vi "Pre Launch Init.vi"(11 "CO2 Actor in":refnum<class "CO2 Actor.lvclass">) -> (0 "error out":errorcluster, 3 "CO2 Actor out":refnum<class "CO2 Actor.lvclass">)   [LabVIEW 2015, in "cRIO-Carbondioxide.lvlib" / "CO2-Actor.lvlib" / "CO2 Actor.lvclass"]
doc: "(<B>Filename</B>: Actor Framework.lvlib:Actor.lvclass:Pre Launch Init.vi)\n\nDefines behavior that occurs after the Launch Actor method is invoked but before the actor's Actor Core method begins running.\n\nThe Pre Launch Init method is guaranteed to finish before the Launch Actor method returns to its caller and before the actor itself receives any messages. Any references that the Pre Launch Init method obtains are guaranteed to have the same lifetime as the actor itself. Any errors that the Pre Launch Init method returns will abort the launch.\n\nBy default, this method does nothing. A descendant class may override it to define behavior."
uses:
  CO2 Actor.lvclass
  cRIO-CO2/Debugger.ctl
  CO2 Actor.lvclass/CO2 Actor.ctl
  <vilib>/ActorFramework/Actor/Actor.lvclass/Actor.ctl
  <vilib>/ActorFramework/Message Enqueuer/Message Enqueuer.lvclass/Message Enqueuer.ctl
  <vilib>/ActorFramework/Message Enqueuer/Init from Existing Queue.vi
  <vilib>/ActorFramework/Message Enqueuer/Enqueue.vi
  <vilib>/ActorFramework/Message Priority Queue/Priority Enqueue.vi
  CO2 Actor Messages/Register Self Msg/Register Self Msg.lvclass
  <vilib>/ActorFramework/Message Enqueuer/Message Enqueuer.lvclass
  <vilib>/ActorFramework/Actor/Actor.lvclass
  cRIO-CO2/cRIO-CO2.lvclass
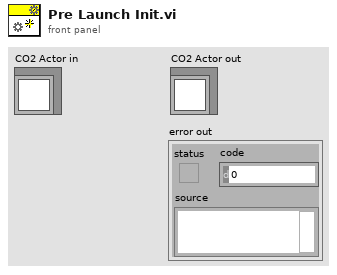
[diagram p1: front panel]
types:
  T1 = typedef "cRIO-Carbondioxide.lvlib/cRIO-CO2.lvlib/cRIO-CO2.lvclass/Debugger.ctl" = cluster{"Log Ref":refnum<vi>, "Debugger Graph Chart Ref":refnum<vi>, "Debug Rng Ref":refnum<vi>}
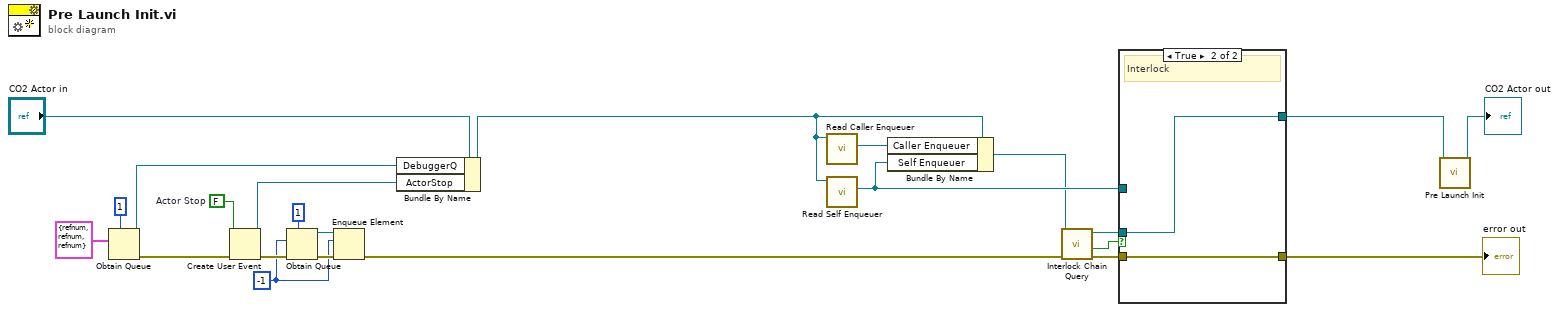
[diagram p0: block diagram]
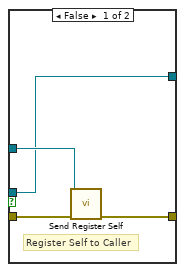
[diagram p2: hidden frame]
diagram:
  w12 = -1 ("Index")
  w3 = FALSE  # Actor Stop
  n1 = Obtain Queue(max queue size (-1, unlimited)=1, element data type=T1 {"Log Ref"=refnum, "Debugger Graph Chart Ref"=refnum, "Debug Rng Ref"=refnum} ("Debuger")) -> (queue out=w21:refnum<queue>, error out=w20:errorcluster)  [unwired: 3 in, 1 out]
  n2 = Create User Event(user event datatype=w3, error in=w20) -> (user event=w19:refnum<user-event>, error out=w16:errorcluster)
  n3 = Obtain Queue(max queue size (-1, unlimited)=1, element data type=w12, error in (no error)=w16) -> (queue out=w13:refnum<queue>, error out=w14:errorcluster)  [unwired: 2 in, 1 out]
  n4 = Enqueue Element(queue=w13, element=w12, error in (no error)=w14) -> (error out=w2:errorcluster)  [unwired: 1 in, 2 out]
  n5 = Bundle By Name(cluster="CO2 Actor in", "DebuggerQ"=w21, "ActorStop"=w19) -> (w1:refnum<class "CO2 Actor.lvclass">)
  n6 = call <vilib>:"Read Caller Enqueuer.vi"("Actor"=w1) -> ("Caller Enqueuer"=w18:refnum<class "Message Enqueuer.lvclass">)  [unwired: 10 in]
  n7 = call <vilib>:"Read Self Enqueuer.vi"("Actor"=w1) -> ("Self Enqueuer"=w9:refnum<class "Message Enqueuer.lvclass">)  [unwired: 10 in]
  n8 = Bundle By Name(cluster=w1, "Caller Enqueuer"=w18, "Self Enqueuer"=w9) -> (w8:refnum<class "CO2 Actor.lvclass">)
  n9 = call-dynamic "Interlock Chain Query.vi"("error in (no error)"=w2, "CO2 Actor in"=w8) -> ("error out"=w11:errorcluster, "Interlock out"=w7:bool, "CO2 Actor out"=w10:refnum<class "CO2 Actor.lvclass">)  [unwired: 6 in, 1 out]
  n10 = case shown="True" w7 {
    tunnel: w11 -> [w27 w29]
    tunnel: [w26 w29] -> w5
    tunnel: w10 -> [w24 w28]
    tunnel: [w24 w28] -> w4
    tunnel: w9 -> [w25 _]
    frame False {
      # "Register Self to Caller"
      n11 = call "Send Register Self.vi"("error in (no error)"=w27, "Message Enqueuer"=w25) -> ("error out"=w26:errorcluster)  [unwired: 8 in, 1 out]
    }
    frame True {
      # "Interlock"
    }
  }
  "error out" <- w5
  n12 = call-parent "Pre Launch Init.vi"("Actor in"=w4) -> ("Actor out"=→"CO2 Actor out":refnum<class "CO2 Actor.lvclass">)  [unwired: 9 in, 1 out]
